vi "DBL_2_STRING_ARRAY.vi"(1 "Insect-data-array":dbl[][](array[numeric])) -> (0 "Insect-data-array":string[][](array[string]))   [LabVIEW 2022 SP3]
doc: "Convertes the double insect-data-array to a sting insect-data-array with headlines"
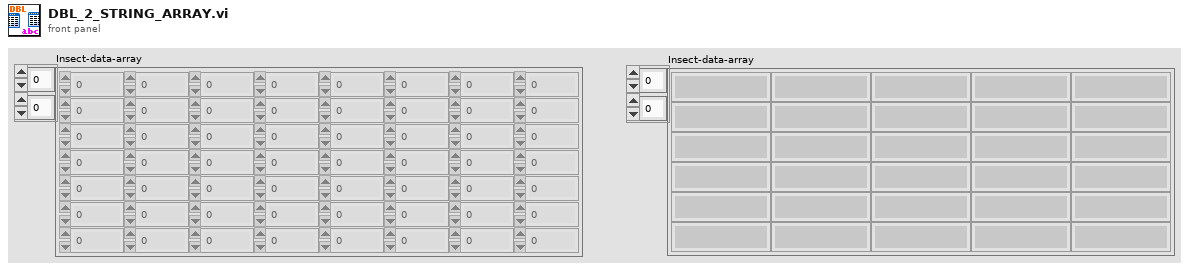
[diagram p1: front panel]
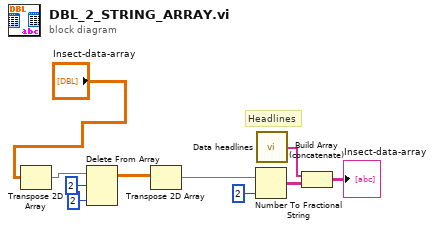
[diagram p0: block diagram]
diagram:
  # "Headlines"
  n1 = Transpose 2D Array(2D array="Insect-data-array") -> (transposed array=w5:dbl[][])
  n2 = Delete From Array(array=w5, length=2, index (row)=2) -> (array with subset deleted=w2:dbl[][])  [unwired: 1 in, 1 out]
  n3 = Transpose 2D Array(2D array=w2) -> (transposed array=w1:dbl[][])
  n4 = Number To Fractional String(number=w1, precision (6)=i16 2) -> (F-format string=w8:string[][])  [unwired: 2 in]
  n5 = call "Data headlines.vi"() -> ("Headlines (vertical array)"=w10:string[])
  n6 = Build Array (concatenate)(w10, w8) -> (→"Insect-data-array":string[][])
